vi "Create Log Specification.vi"(7 "RT Data in":T1={"Device Ref"=18446744073709551615, "Waveforms"=[], "Channels"={"Command Chan Refs"=[], "Command Data Refs"=[], "Command Values"=[], "Status Chan Refs"=[], "Status Data Refs"=[], "Status Values"=[], "System Time"={"System Time"=timestamp(0 s since 1904-01-01), "Data Reference"=0, "Absolute Time Channel Data Ref"=0, "Get Date-Time Channel Data Ref"=0}, "Trigger Chan Refs"=[], "Trigger Data Refs"=[], "Trigger Values"=[]}, "Waveform Logs"=[], "Communication"={"Async Status"=refnum, "Wfm Comm Properties"={"WPL"={"Custom Queue Size"=1, "Use Custom Queue Size?"=FALSE}}, "Shutdown Event"=refnum, "Trigger Event"=refnum, "New File Event"=refnum, "Log Queues"=[], "Async VI Ref"=refnum}, "error"={"status"=FALSE, "code"=0, "source"=""}} {"Device Ref" format="%.0x"; "Channels"."Trigger Data Refs"."Data Reference" format="%.0x"; "Channels"."Trigger Chan Refs" format="%.0x"; "Channels"."System Time"."Get Date-Time Channel Data Ref" format="%.0x"; "Channels"."System Time"."Absolute Time Channel Data Ref" format="%.0x"; "Channels"."System Time"."Channel Data Reference" format="%.0x"; "Channels"."Status Data Refs"."Data Reference" format="%.0x"; "Channels"."Command Data Refs"."Data Reference" format="%.0x"; "Channels"."Status Chan Refs" format="%.0x"; "Channels"."Command Chan Refs" format="%.0x"; "Waveforms"."Waveform Ref in" format="%.0x"; "Waveform Logs"."Node ID" format="%.0x"; "Waveform Logs"."TDMS Error Code"."Data Ref" format="%.0x"; "Waveform Logs"."Missed Samples"."Data Ref" format="%.0x"; "Waveform Logs"."File Status"."Data Ref" format="%.0x"; "Waveform Logs"."Start New File"."Data Ref" format="%.0x"; "Waveform Logs"."Logging Enabled"."Data Ref" format="%.0x"; "Waveform Logs"."Stop Trigger"."Node Data Ref" format="%.0x"; "Waveform Logs"."Stop Trigger"."Node ID" format="%.0x"; "Waveform Logs"."Start Trigger"."Node Data Ref" format="%.0x"; "Waveform Logs"."Start Trigger"."Node ID" format="%.0x"}, 11 "Log Index in":i32) -> (8 "RT Data out":T1={"Device Ref"=18446744073709551615, "Waveforms"=[], "Channels"={"Command Chan Refs"=[], "Command Data Refs"=[], "Command Values"=[], "Status Chan Refs"=[], "Status Data Refs"=[], "Status Values"=[], "System Time"={"System Time"=timestamp(0 s since 1904-01-01), "Data Reference"=0, "Absolute Time Channel Data Ref"=0, "Get Date-Time Channel Data Ref"=0}, "Trigger Chan Refs"=[], "Trigger Data Refs"=[], "Trigger Values"=[]}, "Waveform Logs"=[], "Communication"={"Async Status"=refnum, "Wfm Comm Properties"={"WPL"={"Custom Queue Size"=1, "Use Custom Queue Size?"=FALSE}}, "Shutdown Event"=refnum, "Trigger Event"=refnum, "New File Event"=refnum, "Log Queues"=[], "Async VI Ref"=refnum}, "error"={"status"=FALSE, "code"=0, "source"=""}} {"Device Ref" format="%.0x"; "Channels"."Trigger Data Refs"."Data Reference" format="%.0x"; "Channels"."Trigger Chan Refs" format="%.0x"; "Channels"."System Time"."Get Date-Time Channel Data Ref" format="%.0x"; "Channels"."System Time"."Absolute Time Channel Data Ref" format="%.0x"; "Channels"."System Time"."Channel Data Reference" format="%.0x"; "Channels"."Status Data Refs"."Data Reference" format="%.0x"; "Channels"."Command Data Refs"."Data Reference" format="%.0x"; "Channels"."Status Chan Refs" format="%.0x"; "Channels"."Command Chan Refs" format="%.0x"; "Waveforms"."Waveform Ref in" format="%.0x"; "Waveform Logs"."Node ID" format="%.0x"; "Waveform Logs"."TDMS Error Code"."Data Ref" format="%.0x"; "Waveform Logs"."Missed Samples"."Data Ref" format="%.0x"; "Waveform Logs"."File Status"."Data Ref" format="%.0x"; "Waveform Logs"."Start New File"."Data Ref" format="%.0x"; "Waveform Logs"."Logging Enabled"."Data Ref" format="%.0x"; "Waveform Logs"."Stop Trigger"."Node Data Ref" format="%.0x"; "Waveform Logs"."Stop Trigger"."Node ID" format="%.0x"; "Waveform Logs"."Start Trigger"."Node Data Ref" format="%.0x"; "Waveform Logs"."Start Trigger"."Node ID" format="%.0x"}, 15 "Log Index out":i32)   [LabVIEW 2015, in "Waveform Data Logger Engine.lvlib"]
uses:
  Waveform Data Logger Engine.lvlib
  Types/RT Data.ctl
  <vilib>/NI Veristand/Custom Device API/Custom Device Item Ref.ctl
  Types/Inline Waveform Info.ctl
  <vilib>/NI Veristand/Custom Device API/Waveform Data Reference.ctl
  Classes/Waveforms/Waveform Receive/Associated Log.ctl
  <vilib>/NI Veristand/Custom Device API/Custom Device Waveform DataType.ctl
  Types/Channels.ctl
  <vilib>/NI Veristand/Custom Device API/Block Data Reference.ctl
  <vilib>/NI Veristand/Custom Device API/Data Reference.ctl
  Types/System Time.ctl
  Types/Inline Waveform Log Info.ctl
  Classes/Log File Specifications/Waveform TDMS Log File Specification/Waveform TDMS Log File Specification.lvclass
  Classes/Triggers/Trigger/Trigger.lvclass
  Types/Inline Log Waveform.ctl
  Types/Trigger Settings.ctl
  Types/Log Status.ctl
  Types/Channel.ctl
  Types/Communication.ctl
  Types/Async Status.ctl
  Types/Async State.ctl
  <vilib>/NI Veristand/Custom Device Waveform API/Communication Properties.ctl
  Types/Trigger Event Data.ctl
  Types/Trigger Received.ctl
  Types/New File Event Data.ctl
  Types/Log Queues.ctl
  Classes/Log File Specifications/Log File Specification/Log Specification Type.ctl
  Classes/Log File Specifications/Log File Specification/Log File Specification.lvclass/Log File Specification.ctl
  Shared/Globals/Property Strings.vi
  <vilib>/NI Veristand/Custom Device API/Get Item Property (String).vi
  <vilib>/NI Veristand/Custom Device API/Get Item Property (Path).vi
  <vilib>/NI Veristand/Custom Device API/Get Item Property (U16).vi
  <vilib>/NI Veristand/Custom Device API/Get Item Property (Boolean).vi
  <vilib>/NI Veristand/Custom Device API/Get Item Property (U32).vi
  Classes/Log File Specifications/Log File Specification/Log File Specification.lvclass
  Classes/Log File Specifications/TDMS Log File Specification/TDMS Log File Specification.lvclass
  <vilib>/NI Veristand/Custom Device API/Custom Device API.lvlib
  Shared/Waveform Data Logger Shared.lvlib
  Classes/Waveforms/Waveform Receive/Waveform Receive.lvclass
  <vilib>/NI Veristand/Custom Device Waveform API/NI_VS Custom Device Waveform API.lvlib
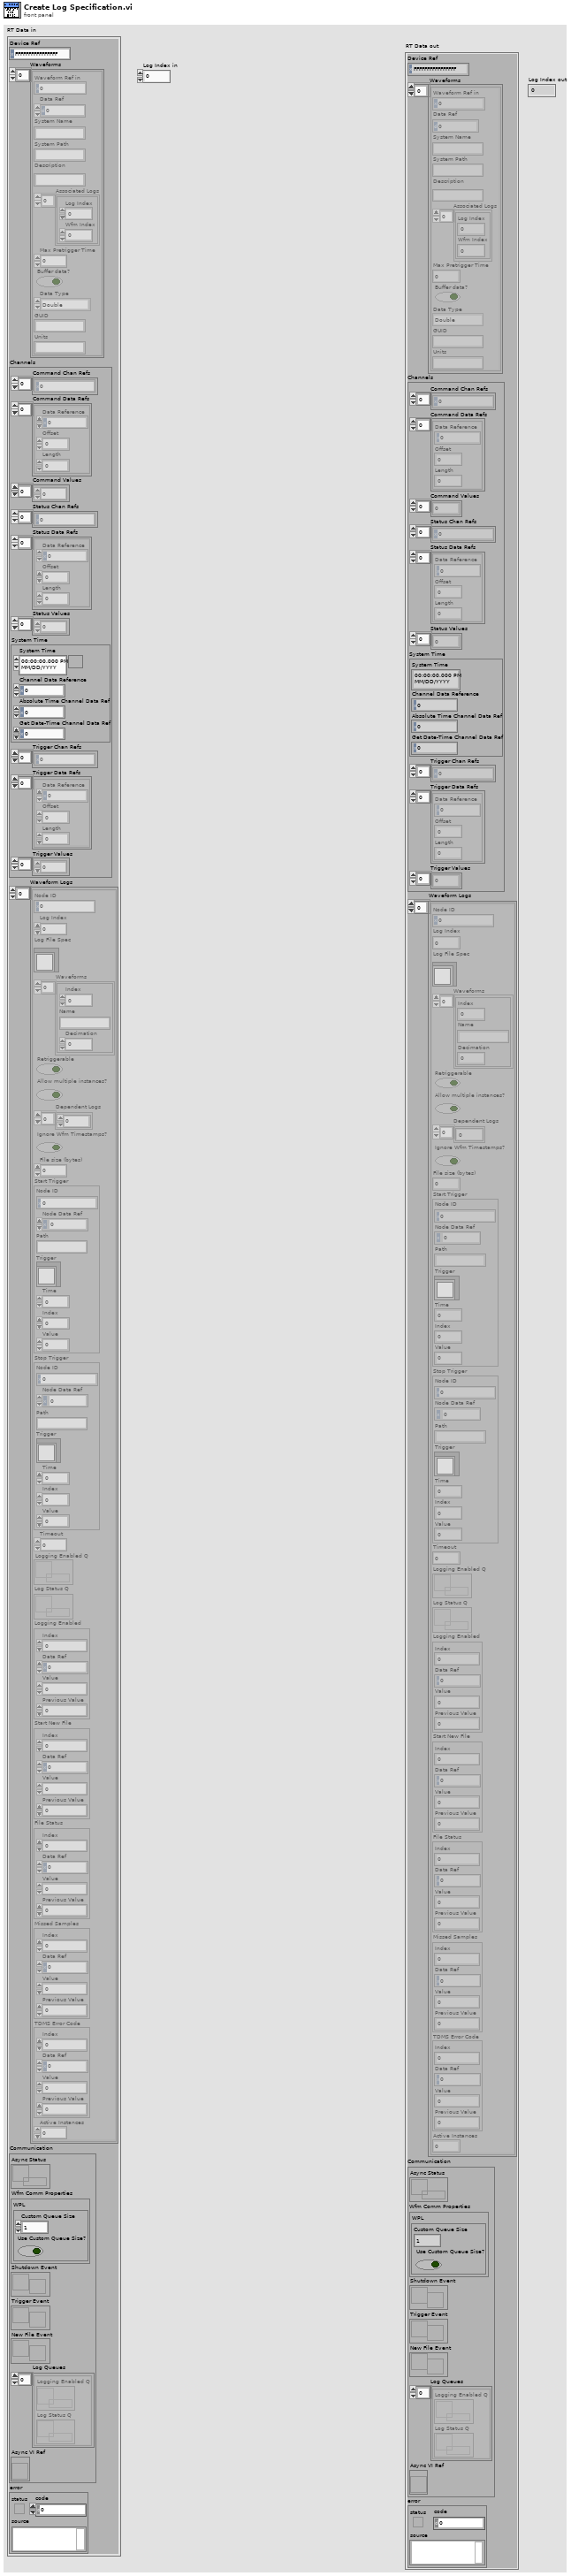
[diagram p1: front panel]
types:
  T1 = typedef "Waveform Data Logger Engine.lvlib/RT Data.ctl" = cluster{"Device Ref":T2, "Waveforms":T3[], "Channels":T7, "Waveform Logs":T11[], "Communication":T15, "error":errorcluster}
  T2 = typedef "Custom Device API.lvlib/Custom Device Item Ref.ctl" = u64
  T3 = typedef "Waveform Data Logger Engine.lvlib/Inline Waveform Info.ctl" = cluster{"Waveform Ref in":T2, "Data Ref":T4, "System Name":string, "System Path":string, "Description":string, "Associated Logs":T5[], "Max Pretrigger Time":dbl, "Buffer data?":bool, "Data Type":T6, "GUID":string, "Units":string}
  T4 = typedef "Custom Device API.lvlib/Waveform Data Reference.ctl" = i32
  T5 = typedef "Waveform Receive.lvclass/Associated Log.ctl" = cluster{"Log Index":i32, "Wfm Index":i32}
  T6 = typedef "Custom Device API.lvlib/Custom Device Waveform DataType.ctl" = enum16{"Double", "Complex Double"}
  T7 = typedef "Waveform Data Logger Engine.lvlib/Channels.ctl" = cluster{"Command Chan Refs":T2[], "Command Data Refs":T8[], "Command Values":dbl[], "Status Chan Refs":T2[], "Status Data Refs":T8[], "Status Values":dbl[], "System Time":T10, "Trigger Chan Refs":T2[], "Trigger Data Refs":T8[], "Trigger Values":dbl[]}
  T8 = typedef "Custom Device API.lvlib/Block Data Reference.ctl" = cluster{"Data Reference":T9, "Offset":u64, "Length":u64}
  T9 = typedef "Custom Device API.lvlib/Data Reference.ctl" = i32
  T10 = typedef "Waveform Data Logger Engine.lvlib/System Time.ctl" = cluster{"System Time":timestamp, "Data Reference":T9, "Absolute Time Channel Data Ref":T9, "Get Date-Time Channel Data Ref":T9}
  T11 = typedef "Waveform Data Logger Engine.lvlib/Inline Waveform Log Info.ctl" = cluster{"Node ID":T2, "Log Index":i32, "Log File Spec":refnum<class "Waveform TDMS Log File Specification.lvclass">, "Waveforms":T12[], "Retriggerable":bool, "Allow multiple instances?":bool, "Dependent Logs":i32[], "Ignore Wfm Timestamps?":bool, "File size (bytes)":i64, "Start Trigger":T13, "Stop Trigger":T13, "Timeout":dbl, "Logging Enabled Q":refnum<queue>, "Log Status Q":refnum<queue>, "Logging Enabled":T14, "Start New File":T14, "File Status":T14, "Missed Samples":T14, "TDMS Error Code":T14, "Active Instances":i32}
  T12 = typedef "Waveform Data Logger Engine.lvlib/Inline Log Waveform.ctl" = cluster{"Index":i32, "Name":string, "Decimation":u32}
  T13 = typedef "Waveform Data Logger Engine.lvlib/Trigger Settings.ctl" = cluster{"Node ID":T2, "Node Data Ref":i32, "Path":string, "Trigger":refnum<class "Trigger.lvclass">, "Time":dbl, "Index":i32, "Value":dbl}
  T14 = typedef "Waveform Data Logger Engine.lvlib/Channel.ctl" = cluster{"Index":i32, "Data Ref":T9, "Value":dbl, "Previous Value":dbl}
  T15 = typedef "Waveform Data Logger Engine.lvlib/Communication.ctl" = cluster{"Async Status":refnum<queue>, "Wfm Comm Properties":T16, "Shutdown Event":refnum<user-event>, "Trigger Event":refnum<user-event>, "New File Event":refnum<user-event>, "Log Queues":T17[], "Async VI Ref":refnum<vi>}
  T16 = typedef "NI_VS Custom Device Waveform API.lvlib/Communication Properties.ctl" = cluster{"WPL":cluster{"Custom Queue Size":i32, "Use Custom Queue Size?":bool}}
  T17 = typedef "Waveform Data Logger Engine.lvlib/Log Queues.ctl" = cluster{"Logging Enabled Q":refnum<queue>, "Log Status Q":refnum<queue>}
  T18 = typedef "Log File Specification.lvclass/Log Specification Type.ctl" = enum16{"Default", "TDMS", "Text", "Waveform TDMS"}
  T19 = typedef "Custom Device API.lvlib/Custom Device Item Info.ctl" = cluster{"Name":string, "Is Channel":bool, "GUID":string, "Is Waveform":bool}
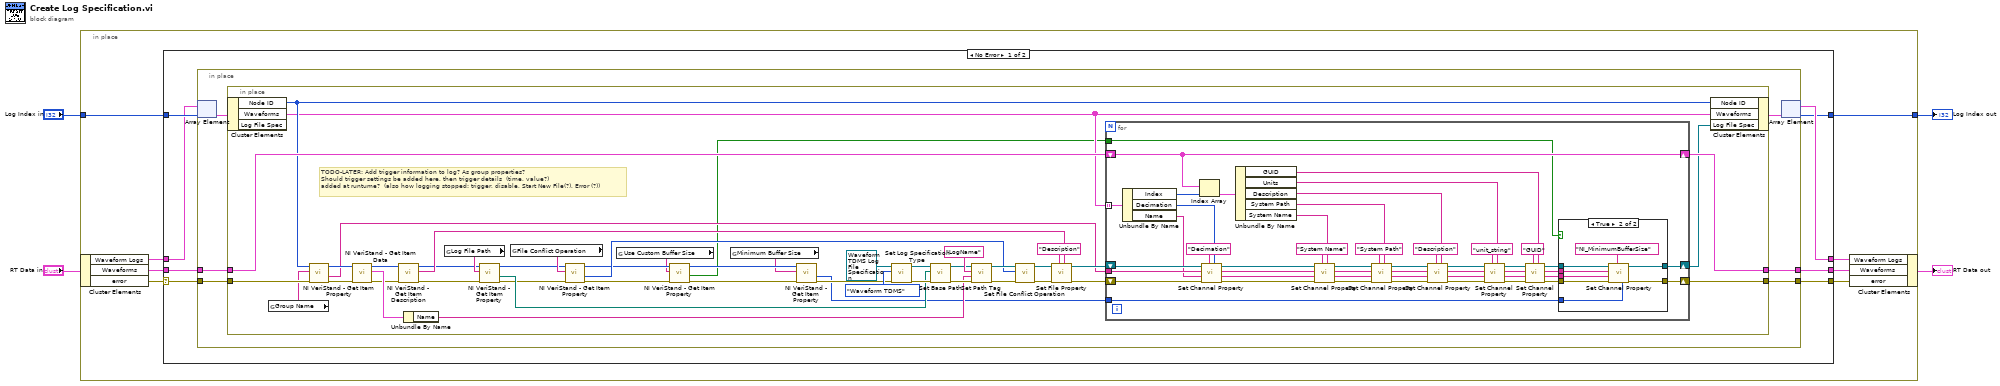
[diagram p0: block diagram]
diagram:
  n1 = in-place {
    in-place-border: "Log Index in" -> [w9]
    in-place-border: [w6] -> w2
    n2 = in-place-cluster #1("RT Data in") -> ("Waveform Logs"=w8:T11[], "Waveforms"=w11:T3[], "error"=w5:errorcluster)
    n3 = case shown="No Error" w5 {
      selector: w5 -> [w13 w132]
      tunnel: [w20 w132] -> w12
      tunnel: w11 -> [w19 w133]
      tunnel: [w18 w133] -> w10
      tunnel: w9 -> [w17 w135]
      tunnel: w8 -> [w16 w134]
      tunnel: [w15 w134] -> w7
      tunnel: [w14 w135] -> w6
      frame No Error {
        n4 = in-place {
          in-place-border: w13 -> [w26]
          in-place-border: [w25] -> w20
          in-place-border: w19 -> [w24]
          in-place-border: [w23] -> w18
          n5 = in-place-array #2(w16, w17) -> (w22:T11)
          n6 = in-place {
            in-place-border: w26 -> [w73]
            in-place-border: [w72] -> w25
            in-place-border: w24 -> [w71]
            in-place-border: [w70] -> w23
            # "TODO-LATER: Add trigger information to log? As group properties?\nShould trigger settings be added here, then trigger details  (time, value?) \nadded at runtume?  (also how logging stopped: trigger, disable, Start New File(?), Error (?))"
            n7 = in-place-cluster #3(w22) -> ("Node ID"=w69:T2, "Waveforms"=w68:T12[])  [unwired: 1 out]
            n8 = global read "Property Strings.vi" "Group Name"() -> (w43:string)
            n9 = call-poly <vilib>:"NI VeriStand - Get Item Property.vi"("error in (no error)"=w73, "Property Name"=w43, "Item Ref in"=w69) -> ("error out"=w42:errorcluster, "Value"=w40:string, "Item Ref out"=w41:T2)  [unwired: 1 in, 5 out]
            n10 = call <vilib>:"NI VeriStand - Get Item Data.vi"("error in (no error)"=w42, "Item Ref in"=w41) -> ("error out"=w47:errorcluster, "Item Info"=w51:T19, "Item Ref out"=w48:T2)  [unwired: 7 out]
            n11 = call <vilib>:"NI VeriStand - Get Item Description.vi"("error in (no error)"=w47, "Item Ref in"=w48) -> ("error out"=w44:errorcluster, "Description"=w46:string, "Item Ref out"=w45:T2)  [unwired: 6 in, 1 out]
            n12 = Unbundle By Name(w51) -> ("Name"=w49:string)
            n13 = global read "Property Strings.vi" "Log File Path"() -> (w52:string)
            n14 = call-poly <vilib>:"NI VeriStand - Get Item Property.vi"("error in (no error)"=w44, "Property Name"=w52, "Item Ref in"=w45) -> ("error out"=w37:errorcluster, "Value"=w50:path, "Item Ref out"=w38:T2)  [unwired: 1 in, 5 out]
            n15 = global read "Property Strings.vi" "File Conflict Operation"() -> (w39:string)
            n16 = call-poly <vilib>:"NI VeriStand - Get Item Property.vi"("error in (no error)"=w37, "Property Name"=w39, "Item Ref in"=w38) -> ("error out"=w35:errorcluster, "Value"=w36:u16, "Item Ref out"=w34:T2)  [unwired: 1 in, 5 out]
            n17 = global read "Property Strings.vi" "Use Custom Buffer Size"() -> (w33:string)
            n18 = call-poly <vilib>:"NI VeriStand - Get Item Property.vi"("error in (no error)"=w35, "Property Name"=w33, "Item Ref in"=w34) -> ("error out"=w31:errorcluster, "Value"=w28:bool, "Item Ref out"=w32:T2)  [unwired: 1 in, 5 out]
            n19 = global read "Property Strings.vi" "Minimum Buffer Size"() -> (w30:string)
            n20 = call-poly <vilib>:"NI VeriStand - Get Item Property.vi"("error in (no error)"=w31, "Property Name"=w30, "Item Ref in"=w32) -> ("error out"=w29:errorcluster, "Value"=w27:u32)  [unwired: 1 in, 6 out]
            n21 = call "Set Log Specification Type.vi"("error in (no error)"=w29, "Log Specification Type"=Log_Specification_Type."Waveform TDMS", "Log File Specification in"=refnum<class "Waveform TDMS Log File Specification.lvclass"> refnum ("Waveform Data Logger Engine.lvlib:Waveform TDMS Log File Specification.lvclass")) -> ("error out"=w64:errorcluster, "Log File Specification out"=w63:refnum<class "Waveform TDMS Log File Specification.lvclass">)  [unwired: 7 in]
            n22 = call "Set Base Path.vi"("error in (no error)"=w64, "Base Path"=w50, "Log File Specification in"=w63) -> ("error out"=w53:errorcluster, "Log File Specification out"=w56:refnum<class "Waveform TDMS Log File Specification.lvclass">)  [unwired: 7 in]
            n23 = call "Set Path Tag.vi"("error in (no error)"=w53, "Tag Value"=w49, "Tag Name"="LogName", "Log File Specification in"=w56) -> ("error out"=w54:errorcluster, "Log File Specification out"=w55:refnum<class "Waveform TDMS Log File Specification.lvclass">)  [unwired: 6 in]
            n24 = call "Set File Conflict Operation.vi"("error in (no error)"=w54, "File Conflict Operation"=w36, "Log File Specification in"=w55) -> ("error out"=w61:errorcluster, "Log File Specification out"=w60:refnum<class "Waveform TDMS Log File Specification.lvclass">)  [unwired: 7 in]
            n25 = call "Set File Property.vi"("Value"=w46, "Name"="Description", "error in (no error)"=w61, "TDMS Log File Specification in"=w60) -> ("error out"=w58:errorcluster, "TDMS Log File Specification out"=w59:refnum<class "Waveform TDMS Log File Specification.lvclass">)  [unwired: 6 in]
            n26 = for {
              shift-right: [w76] -> w67
              shift-left: w59 -> [w113]
              shift-right: [w77] -> w72
              shift-left: w58 -> [w114]
              tunnel: w40 -> [w112]
              tunnel: w68 -> [w116] mode=indexing
              shift-right: [w115] -> w70
              shift-left: w71 -> [w115]
              tunnel: w28 -> [w74]
              tunnel: w27 -> [w75]
              n27 = Unbundle By Name(w116) -> ("Index"=w110:i32, "Decimation"=w109:u32, "Name"=w111:string)
              n28 = Index Array(array=w115, index=w110) -> (element=w108:T3)
              n29 = call "Set Channel Property.vi"("Value"=w109, "Name"="Decimation", "error in (no error)"=w114, "Channel Name in"=w111, "Group Name in"=w112, "TDMS Log File Specification in"=w113) -> ("error out"=w86:errorcluster, "Channel Name out"=w87:string, "Group Name out"=w88:string, "TDMS Log File Specification out"=w89:refnum<class "Waveform TDMS Log File Specification.lvclass">)  [unwired: 2 in]
              n30 = Unbundle By Name(w108) -> ("GUID"=w102:string, "Units"=w103:string, "Description"=w104:string, "System Path"=w105:string, "System Name"=w106:string)
              n31 = call "Set Channel Property.vi"("Value"=w106, "Name"="System Name", "error in (no error)"=w86, "Channel Name in"=w87, "Group Name in"=w88, "TDMS Log File Specification in"=w89) -> ("error out"=w82:errorcluster, "Channel Name out"=w83:string, "Group Name out"=w84:string, "TDMS Log File Specification out"=w85:refnum<class "Waveform TDMS Log File Specification.lvclass">)  [unwired: 2 in]
              n32 = call "Set Channel Property.vi"("Value"=w105, "Name"="System Path", "error in (no error)"=w82, "Channel Name in"=w83, "Group Name in"=w84, "TDMS Log File Specification in"=w85) -> ("error out"=w90:errorcluster, "Channel Name out"=w91:string, "Group Name out"=w92:string, "TDMS Log File Specification out"=w93:refnum<class "Waveform TDMS Log File Specification.lvclass">)  [unwired: 2 in]
              n33 = call "Set Channel Property.vi"("Value"=w104, "Name"="Description", "error in (no error)"=w90, "Channel Name in"=w91, "Group Name in"=w92, "TDMS Log File Specification in"=w93) -> ("error out"=w97:errorcluster, "Channel Name out"=w96:string, "Group Name out"=w95:string, "TDMS Log File Specification out"=w94:refnum<class "Waveform TDMS Log File Specification.lvclass">)  [unwired: 2 in]
              n34 = call "Set Channel Property.vi"("Value"=w103, "Name"="unit_string", "error in (no error)"=w97, "Channel Name in"=w96, "Group Name in"=w95, "TDMS Log File Specification in"=w94) -> ("error out"=w98:errorcluster, "Channel Name out"=w99:string, "Group Name out"=w100:string, "TDMS Log File Specification out"=w101:refnum<class "Waveform TDMS Log File Specification.lvclass">)  [unwired: 2 in]
              n35 = call "Set Channel Property.vi"("Value"=w102, "Name"="GUID", "error in (no error)"=w98, "Channel Name in"=w99, "Group Name in"=w100, "TDMS Log File Specification in"=w101) -> ("error out"=w81:errorcluster, "Channel Name out"=w78:string, "Group Name out"=w79:string, "TDMS Log File Specification out"=w80:refnum<class "Waveform TDMS Log File Specification.lvclass">)  [unwired: 2 in]
              n36 = case shown="True" w74 {
                tunnel: w81 -> [w122 w131]
                tunnel: w80 -> [w123 w130]
                tunnel: w79 -> [_ w129]
                tunnel: w78 -> [_ w128]
                tunnel: [w122 w127] -> w77
                tunnel: [w123 w126] -> w76
                tunnel: w75 -> [_ w124]
                frame False {
                }
                frame True {
                  n37 = call "Set Channel Property.vi"("Value"=w124, "Name"="NI_MinimumBufferSize", "error in (no error)"=w131, "Channel Name in"=w128, "Group Name in"=w129, "TDMS Log File Specification in"=w130) -> ("error out"=w127:errorcluster, "TDMS Log File Specification out"=w126:refnum<class "Waveform TDMS Log File Specification.lvclass">)  [unwired: 2 in, 2 out]
                }
              }
            }
            n38 = in-place-cluster #3("Node ID"=w69, "Waveforms"=w68, "Log File Spec"=w67) -> (w21:T11)
          }
          n39 = in-place-array #2(w21) -> (w15:T11[], w14:i32)
        }
      }
      frame Error {
      }
    }
    n40 = in-place-cluster #1("Waveform Logs"=w7, "Waveforms"=w10, "error"=w12) -> (→"RT Data out":T1)
  }
  "Log Index out" <- w2
